vi "StartStopMesaurement.vi"() -> ()   [LabVIEW 2013]
panel:
  in  "Boolean":bool
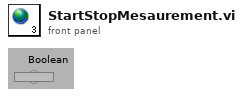
[diagram p1: front panel]
diagram:
